vi "verifyImageLoadAndResize.vi"() -> ()   [LabVIEW 2013]
uses:
  System.Windows.Forms
  System.Drawing
panel:
  in  "Path":path=path "C:/Users/Mike/Desktop/32738A6E00000578-3504412-image-a-6_1458654517341.jpg"
  in  "PictureBox":refnum<k24>(container)
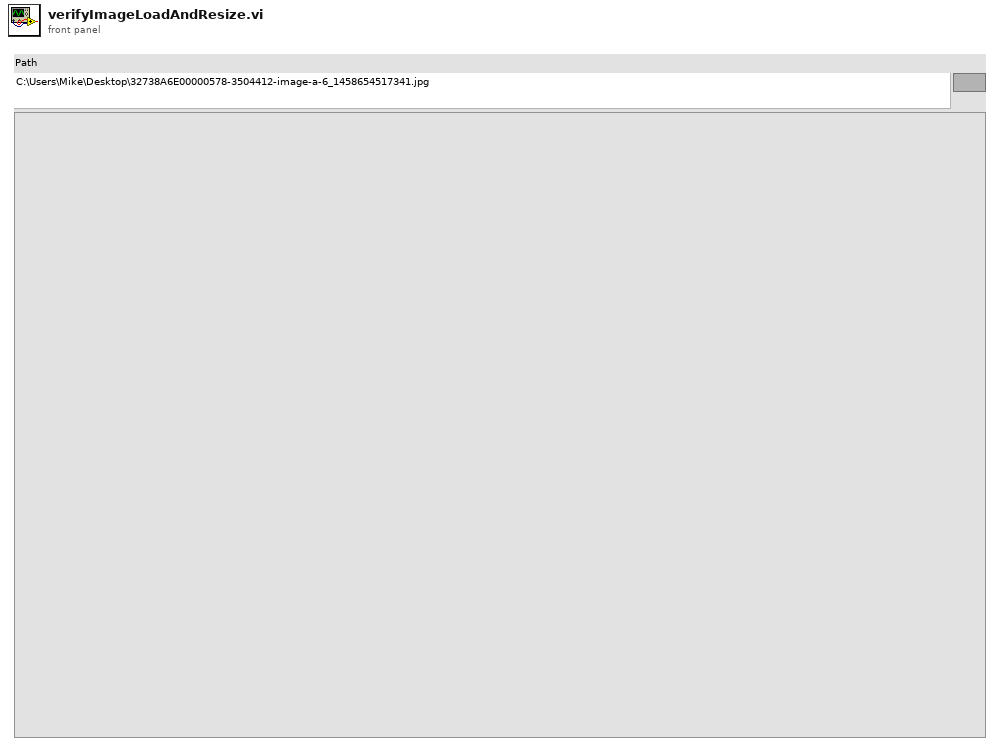
[diagram p1: front panel]
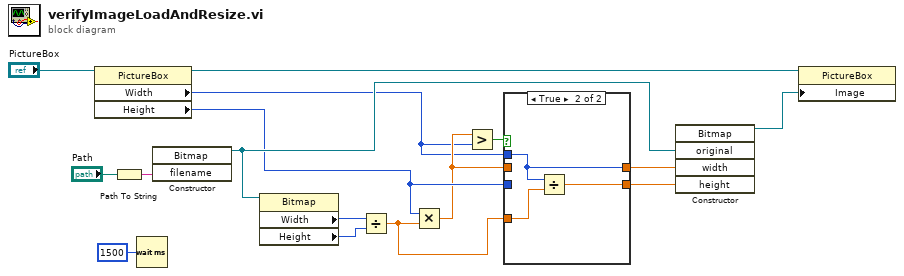
[diagram p0: block diagram]
diagram:
  n1 = property class="PictureBox"(reference="PictureBox") -> (reference out=w10:refnum<k24>, "Width"=w2:i32, "Height"=w6:i32)  [unwired: 1 in, 1 out]
  n2 = Path To String(path="Path") -> (string=w14:string)
  n3 = Wait (ms)(milliseconds to wait=u32 1500) -> ()  [unwired: 1 out]
  n4 = constructor class="Bitmap"("filename"=w14) -> (reference out=w9:refnum<k24>)  [unwired: 3 in, 3 out]
  n5 = property class="Bitmap"(reference=w9) -> ("Width"=w13:i32, "Height"=w12:i32)  [unwired: 1 in, 2 out]
  n6 = Divide(x=w13, y=w12) -> (x/y=w3:dbl)
  n7 = Multiply(x=w6, y=w3) -> (x*y=w4:dbl)
  n8 = Greater?(x=w4, y=w2) -> (0:w8:bool)
  n9 = case shown="True" w8 {
    tunnel: w4 -> [w18 _]
    tunnel: [w18 w19] -> w7
    tunnel: w6 -> [w17 _]
    tunnel: [w17 w20] -> w5
    tunnel: w3 -> [_ w21]
    tunnel: w2 -> [_ w19]
    frame False {
    }
    frame True {
      n10 = Divide(x=w19, y=w21) -> (x/y=w20:dbl)
    }
  }
  n11 = constructor class="Bitmap"("original"=w9, "width"=w7, "height"=w5) -> (reference out=w11:refnum<k24>)  [unwired: 3 in, 5 out]
  n12 = property class="PictureBox"(reference=w10, "Image"=w11) -> ()  [unwired: 1 in, 2 out]
